vi "Quadratic method RT.vi"(8 "Next Amplitude":dbl, 9 "Max Amplitude":dbl, 10 "Max bin":i32, 11 "Prev Amplitude":dbl) -> (3 "Bin":dbl)   [LabVIEW 2014]
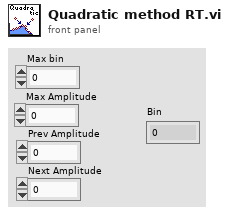
[diagram p1: front panel]
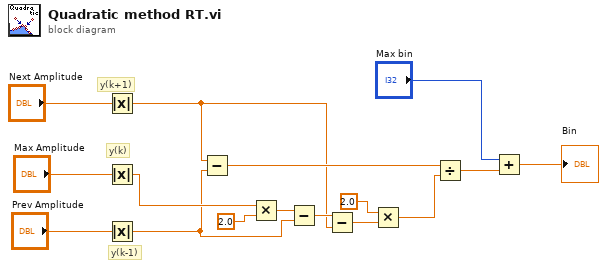
[diagram p0: block diagram]
diagram:
  # "y(k-1)"
  # "y(k+1)"
  # "y(k)"
  n1 = Absolute Value(x="Next Amplitude") -> (abs(x)=w10:dbl)
  n2 = Absolute Value(x="Max Amplitude") -> (abs(x)=w15:dbl)
  n3 = Absolute Value(x="Prev Amplitude") -> (abs(x)=w12:dbl)
  n4 = Subtract(x=w10, y=w12) -> (x-y=w16:dbl)
  n5 = Multiply(x=w15, y=2.0) -> (x*y=w13:dbl)
  n6 = Subtract(x=w13, y=w12) -> (x-y=w11:dbl)
  n7 = Subtract(x=w11, y=w10) -> (x-y=w9:dbl)
  n8 = Multiply(x=2.0, y=w9) -> (x*y=w7:dbl)
  n9 = Divide(x=w16, y=w7) -> (x/y=w6:dbl)
  n10 = Add(x="Max bin", y=w6) -> (x+y=→"Bin":dbl)
